vi "PID_globals.vi"() -> ()   [LabVIEW 2009]
panel:
  in  "Derivative":dbl[](array[numeric])=[0.9, 2.25, 0.9]
  in  "Integral":i32[](array[numeric])=[12, 65, 12]
  in  "PropBand":i32[](array[numeric])=[47, 65, 47]
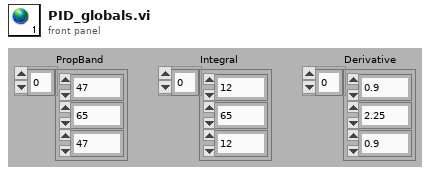
[diagram p1: front panel]
diagram:
